vi "Set Prism Position.vi"(8 "error in (no error)":errorcluster, 10 "Prism Position":enum16{"Removed", "Inserted"}(ring), 11 "TE2000 in":refnum<class "Eclipse TI.lvclass">) -> (0 "error out":errorcluster, 3 "TE2000 out":refnum<class "Eclipse TI.lvclass">)   [LabVIEW 2015, in "Eclipse TI.lvlib" / "Eclipse TI.lvclass"]
uses:
  Eclipse TI.lvclass
  Eclipse TI.lvclass/Eclipse TI.ctl
  <vilib>/Utility/error.llb/Error Cluster From Error Code.vi
  <vilib>/ErrorRing/Error Ring.xnode
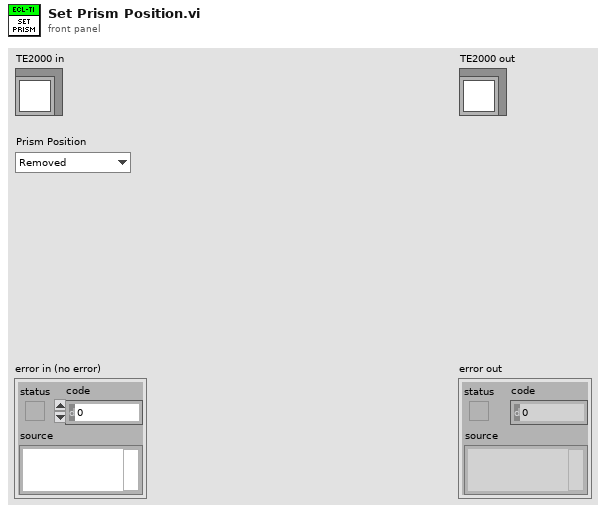
[diagram p1: front panel]
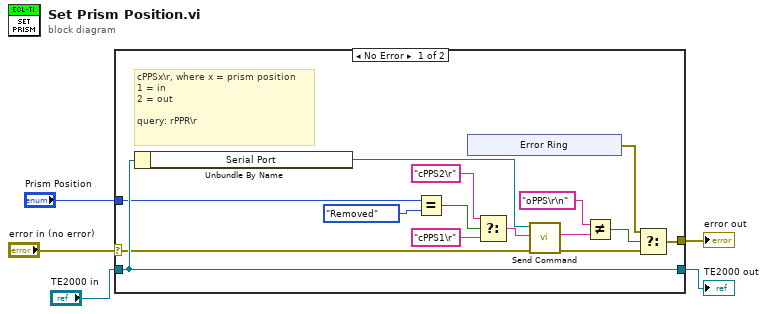
[diagram p0: block diagram]
diagram:
  n1 = case shown="No Error" "error in (no error)" {
    selector: "error in (no error)" -> [w13 w27]
    tunnel: [w7 w27] -> w4
    tunnel: [w20 w26] -> w2
    tunnel: "TE2000 in" -> [w20 w26]
    tunnel: "Prism Position" -> [w19 _]
    frame No Error {
      # "cPPSx\\r, where x = prism position\n1 = in\n2 = out\n\nquery: rPPR\\r"
      n2 = Unbundle By Name(w20) -> ("Serial Port"=w6:refnum<visa-resource-name>)
      n3 = Equal?(x=w19, y=enum16{"Removed", "Inserted"}."Removed") -> (x = y?=w17:bool)
      n4 = xnode "Error Ring"() -> ("error out"=w8:errorcluster)
      n5 = Select(t="cPPS2\r", s=w17, f="cPPS1\r") -> (s? t:f=w16:string)
      n6 = call "Send Command.vi"("error in (no error)"=w13, "Command"=w16, "Serial Port In"=w6) -> ("error out"=w9:errorcluster, "Response"=w12:string)  [unwired: 6 in, 1 out]
      n7 = Not Equal?(x="oPPS\r\n", y=w12) -> (x != y?=w10:bool)
      n8 = Select(t=w8, s=w10, f=w9) -> (s? t:f=w7:errorcluster)
    }
    frame Error {
    }
  }
  "error out" <- w4
  "TE2000 out" <- w2
